vi "windows.vi"() -> ()   [LabVIEW 2009]
uses:
  <vilib>/Analysis/4window.llb/Kaiser-Bessel Window (DBL).vi
  <vilib>/Analysis/NI_AALPro.lvlib
panel:
  in  "stop":bool
  in  "beta":dbl format="%0.2f"
  in  "f=final value":dbl
  in  "Window Type":T1(ring)
  out "Window":dbl[](graph)=[0.0, 0.003942649342761062, 0.015708419435684462, 0.03511175705587427, 0.06184665997806821, 0.09549150281252627, 0.13551568628929422, 0.18128800512565513, 0.23208660251050173, 0.28711035421746367, 0.3454915028125263, 0.40630934270713764, 0.46860474023534326, 0.5313952597646567, 0.5936906572928623, 0.6545084971874735, 0.7128896457825363, 0.7679133974894985, 0.8187119948743449, 0.8644843137107057, 0.9045084971874737, 0.9381533400219317, 0.9648882429441257, 0.9842915805643155, 0.9960573506572389, 1.0, 0.996057350657239, 0.9842915805643155, 0.9648882429441257, 0.9381533400219317, 0.904508497187474, 0.8644843137107059, 0.8187119948743448, 0.7679133974894982, 0.7128896457825361, 0.6545084971874737, 0.5936906572928623, 0.5313952597646566, 0.4686047402353436, 0.40630934270713787, 0.3454915028125264, 0.2871103542174641, 0.23208660251050162, 0.18128800512565535, 0.1355156862892944, 0.09549150281252633, 0.06184665997806843, 0.03511175705587427, 0.015708419435684517, 0.0039426493427611176]
  in  "N":dbl=50.0
  # "Program developed by Indranil Sinharoy"
  # "Exponential window"
  # "Kaiser-Bessel"
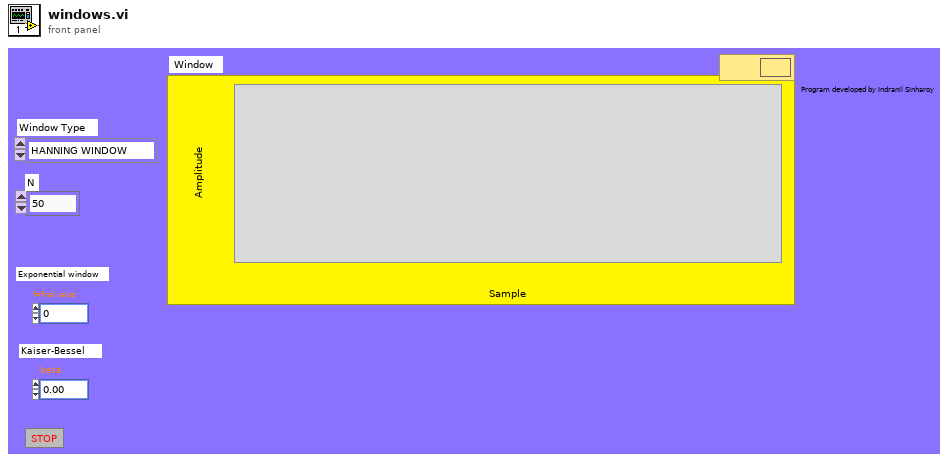
[diagram p1: front panel]
types:
  T1 = enum16{"HANNING WINDOW", "HAMMING WINDOW", "FLAT TOP WINDOW", "RECTANGULAR", "TRIANGLE", "EXPONENTIAL WINDOW", "KAISER-BESSEL WINDOW"}
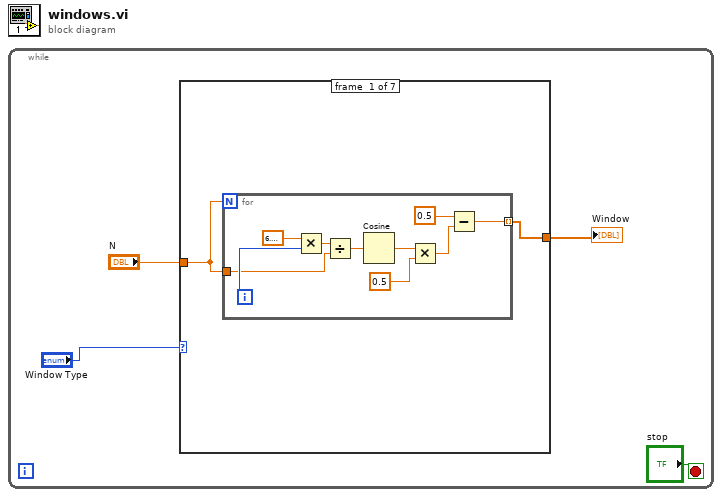
[diagram p0: block diagram]
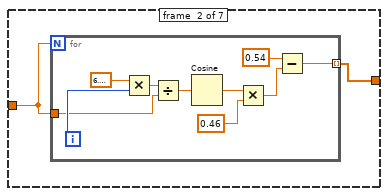
[diagram p2: hidden frame]
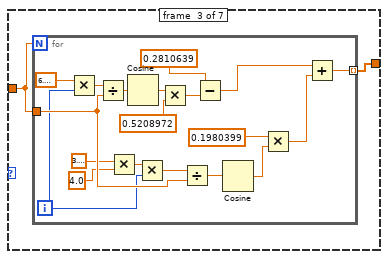
[diagram p3: hidden frame]
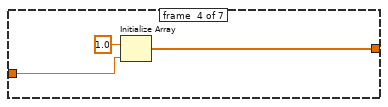
[diagram p4: hidden frame]
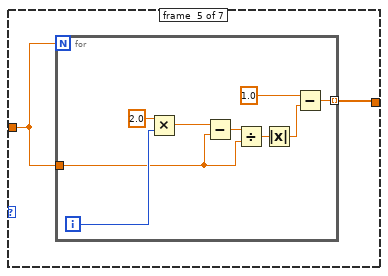
[diagram p5: hidden frame]
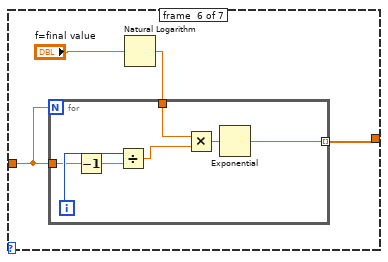
[diagram p6: hidden frame]
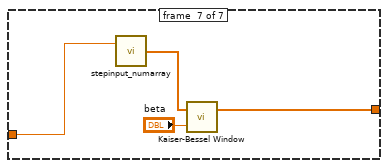
[diagram p7: hidden frame]
diagram:
  n1 = while {
    stop <- "stop" stop-if-true
    n2 = case shown="\"KAISER-BESSEL WINDOW\"" "Window Type" {
      tunnel: [w5 w17 w29 w50 w53 w65 w78] -> w4
      tunnel: "N" -> [w6 w18 w30 w52 w54 w64 w77]
      frame #0 {
        n3 = for {
          N: w6 -> [_]
          tunnel: w6 -> [w12]
          tunnel: [w7] -> w5 mode=indexing
          i -> [w14]
          n4 = Multiply(x=6.283185307179586, y=w14) -> (x*y=w13:dbl)
          n5 = Divide(x=w13, y=w12) -> (x/y=w11:dbl)
          n6 = Cosine(x=w11) -> (cos(x)=w10:dbl)
          n7 = Multiply(x=w10, y=0.5) -> (x*y=w8:dbl)
          n8 = Subtract(x=0.5, y=w8) -> (x-y=w7:dbl)
        }
      }
      frame #1 {
        n9 = for {
          N: w18 -> [_]
          tunnel: w18 -> [w24]
          tunnel: [w19] -> w17 mode=indexing
          i -> [w26]
          n10 = Multiply(x=6.283185307179586, y=w26) -> (x*y=w25:dbl)
          n11 = Divide(x=w25, y=w24) -> (x/y=w23:dbl)
          n12 = Cosine(x=w23) -> (cos(x)=w22:dbl)
          n13 = Multiply(x=w22, y=0.46) -> (x*y=w20:dbl)
          n14 = Subtract(x=0.54, y=w20) -> (x-y=w19:dbl)
        }
      }
      frame #2 {
        n15 = for {
          N: w30 -> [_]
          tunnel: w30 -> [w40]
          tunnel: [w31] -> w29 mode=indexing
          i -> [w38]
          n16 = Multiply(x=6.283185307179586, y=w38) -> (x*y=w47:dbl)
          n17 = Divide(x=w47, y=w40) -> (x/y=w46:dbl)
          n18 = Multiply(x=3.141592653589793, y=4.0) -> (x*y=w39:dbl)
          n19 = Cosine(x=w46) -> (cos(x)=w45:dbl)
          n20 = Multiply(x=w39, y=w38) -> (x*y=w41:dbl)
          n21 = Multiply(x=w45, y=0.5208972) -> (x*y=w43:dbl)
          n22 = Divide(x=w41, y=w40) -> (x/y=w35:dbl)
          n23 = Subtract(x=0.2810639, y=w43) -> (x-y=w42:dbl)
          n24 = Cosine(x=w35) -> (cos(x)=w34:dbl)
          n25 = Multiply(x=0.1980399, y=w34) -> (x*y=w32:dbl)
          n26 = Add(x=w42, y=w32) -> (x+y=w31:dbl)
        }
      }
      frame #3 {
        n27 = Initialize Array(1.0 ("element"), w52) -> (w50:dbl[])
      }
      frame #4 {
        n28 = for {
          N: w54 -> [_]
          tunnel: w54 -> [w58]
          tunnel: [w55] -> w53 mode=indexing
          i -> [w61]
          n29 = Multiply(x=2.0, y=w61) -> (x*y=w60:dbl)
          n30 = Subtract(x=w60, y=w58) -> (x-y=w59:dbl)
          n31 = Divide(x=w59, y=w58) -> (x/y=w57:dbl)
          n32 = Absolute Value(x=w57) -> (abs(x)=w56:dbl)
          n33 = Subtract(x=1.0, y=w56) -> (x-y=w55:dbl)
        }
      }
      frame #5 {
        n34 = Natural Logarithm(1:"f=final value") -> (0:w66:dbl)
        n35 = for {
          N: w64 -> [_]
          tunnel: w66 -> [w71]
          tunnel: w64 -> [w73]
          tunnel: [w68] -> w65 mode=indexing
          i -> [w74]
          n36 = Decrement(x=w73) -> (x-1=w72:dbl)
          n37 = Divide(x=w74, y=w72) -> (x/y=w70:dbl)
          n38 = Multiply(x=w71, y=w70) -> (x*y=w69:dbl)
          n39 = Exponential(1:w69) -> (0:w68:dbl)
        }
      }
      frame #6 {
        n40 = call "stepinput_numarray.vi"("Samples"=w77) -> ("OUTPUT ARRAY"=w76:dbl[])  [unwired: 1 in]
        n41 = call-poly <vilib>:"Kaiser-Bessel Window.vi"("beta"="beta", "X"=w76) -> ("Windowed X"=w78:dbl[])  [unwired: 1 out]
      }
    }
    "Window" <- w4
  }
